vi "showrunningvis.vi"() -> ()   [LabVIEW 2012]
doc: "This example checks the execution state of all VIs in memory and displays the names and front panels of running VIs. You can configure it to display only top-level running VIs, only running subVIs, or both. A VI is in the \"Run top level\" state if its Run button was pressed and it hasn't finished executing. A VI is in the \"Running\" state if it is a subVI of a running VI. This VI uses application and VI property nodes to find the VIs in memory and read their execution state. \n \nUse this VI if you receive the \"Quitting will abort all running VIs\" when you try to exit LabVIEW and you have too many VIs to search manually to find out which one is running."
panel:
  in  "Show Back Panels":bool
  out "VIs Found":string[][](table)
  in  "Show Front Panels":bool=TRUE
  # "Select HelpÈShow Context Help and move the cursor over the VI icon to display help for this VI."
  # "This example checks the execution state of all VIs in memory and displays the names and front panels of \ntop level running VIs.  A VI is in the \"Run top level\" state if its Run button was pressed and it hasn't finished executing \nor if it was started through invoking the run vi method. This VI uses application and VI property nodes to find\nthe VIs in memory and read their execution state. \n \nUse this VI if you receive the \"Quitting will abort all running VIs\" when you try to exit LabVIEW \nand you have too many VIs to search manually to find out which one is running."
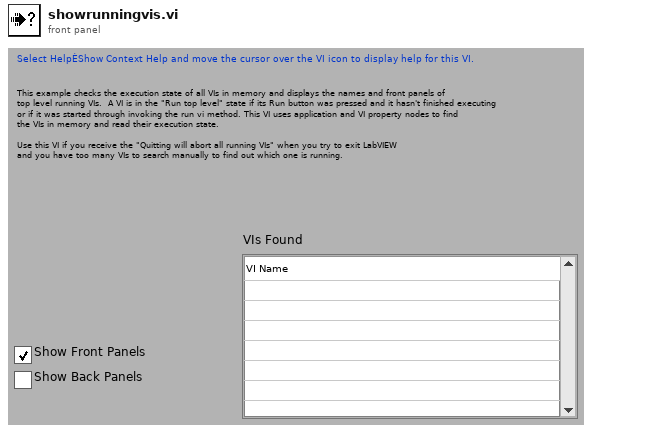
[diagram p1: front panel]
types:
  T1 = enum32{"Bad", "Idle", "Run top level", "Running"}
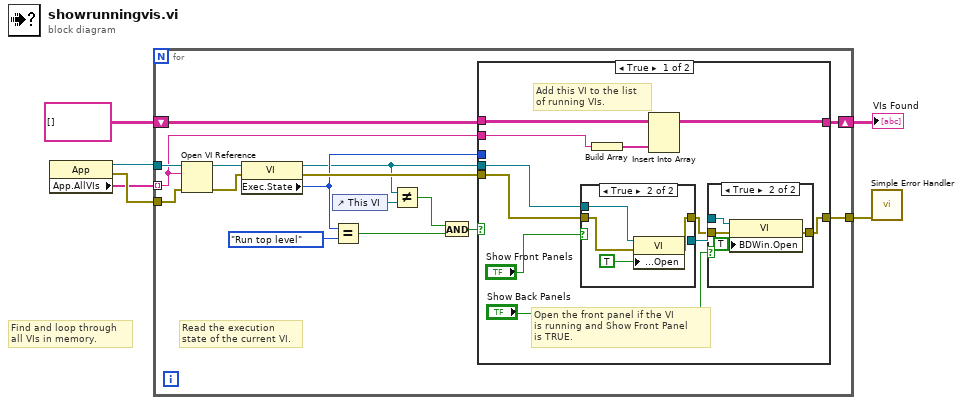
[diagram p0: block diagram]
diagram:
  # "Find and loop through\nall VIs in memory."
  n1 = property class="App"() -> (reference out=w5:refnum<vi>, error out=w6:errorcluster, "App.AllVIs"=w4:string[])  [unwired: 2 in]
  n2 = for {
    tunnel: w4 -> [w16] mode=indexing
    tunnel: w6 -> [w20]
    tunnel: w5 -> [w21]
    shift-right: [w15] -> w1
    shift-left: string[][] [] ("Application:All VIs In Memory") -> [w17]
    tunnel: [w14] -> w2
    # "Read the execution\nstate of the current VI."
    n3 = Open VI Reference(application reference (local)=w21, vi path=w16, error in (no error)=w20) -> (vi reference=w22:refnum<vi>, error out=w19:errorcluster)  [unwired: 3 in]
    n4 = property class="VI"(reference=w22, error in=w19) -> (reference out=w11:refnum<vi>, error out=w18:errorcluster, "Exec.State"=w12:T1)
    n5 = control-ref of="This VI"() -> (w10:refnum<vi>)
    n6 = Equal?(x=w12, y=T1."Run top level" ("Execution:State")) -> (x = y?=w7:bool)
    n7 = Not Equal?(x=w11, y=w10) -> (x != y?=w9:bool)
    n8 = And(x=w9, y=w7) -> (x .and. y?=w8:bool)
    n9 = case shown="True" w8 {
      tunnel: w18 -> [w33 w46]
      tunnel: w11 -> [w27 _]
      tunnel: w17 -> [w32 w47]
      tunnel: w16 -> [w29 _]
      tunnel: [w31 w47] -> w15
      tunnel: [w23 w46] -> w14
      tunnel: w12 -> [_ _]
      frame True {
        # "Add this VI to the list \nof running VIs."
        # "Open the front panel if the VI\nis running and Show Front Panel \nis TRUE."
        n10 = case shown="True" "Show Front Panels" {
          tunnel: w33 -> [w40 w44]
          tunnel: w27 -> [w39 w43]
          tunnel: [w40 w42] -> w24
          tunnel: [w39 w41] -> w25
          frame False {
          }
          frame True {
            n11 = property class="VI"(reference=w43, error in=w44, "Front Panel.Open"=TRUE ("Front Panel Window:Open")) -> (reference out=w41:refnum<vi>, error out=w42:errorcluster)
          }
        }
        n12 = Build Array(w29) -> (w28:string[])
        n13 = Insert Into Array(array=w32, new element=w28) -> (w31:string[][])  [unwired: 2 in]
        n14 = case shown="True" "Show Back Panels" {
          tunnel: w25 -> [_ w38]
          tunnel: w24 -> [w34 w36]
          tunnel: [w34 w35] -> w23
          frame False {
          }
          frame True {
            n15 = property class="VI"(reference=w38, error in=w36, "BDWin.Open"=TRUE ("Block Diagram Window:Open")) -> (error out=w35:errorcluster)  [unwired: 1 out]
          }
        }
      }
      frame False {
      }
    }
  }
  "VIs Found" <- w1
  n16 = call <vilib>:"Simple Error Handler.vi"("error in (no error)"=w2) -> ()  [unwired: 4 in, 5 out]
